vi "Frame Set Sound.vi"(8 "error in (no error)":errorcluster, 10 "Sound":string, 11 "IDE simple in":refnum<class "LF2R IDE.lvclass">) -> (0 "error out":errorcluster, 3 "IDE simple out":refnum<class "LF2R IDE.lvclass">)   [LabVIEW 2018, in "LF2R IDE.lvlib" / "LF2R IDE.lvclass"]
uses:
  LF2R IDE.lvclass
  LF2R IDE.lvclass/LF2R IDE.ctl
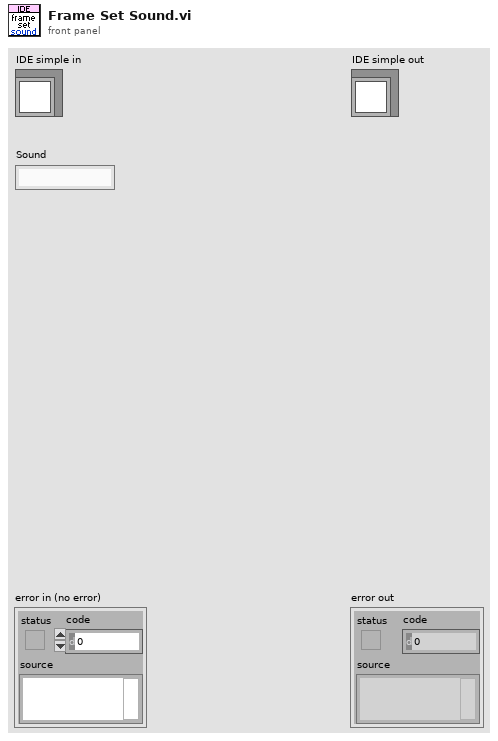
[diagram p1: front panel]
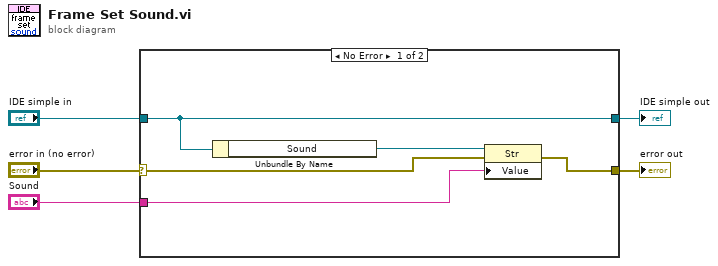
[diagram p0: block diagram]
diagram:
  n1 = case shown="No Error" "error in (no error)" {
    selector: "error in (no error)" -> [w6 w12]
    tunnel: [w7 w12] -> w4
    tunnel: [w10 w11] -> w2
    tunnel: "IDE simple in" -> [w10 w11]
    tunnel: "Sound" -> [w8 _]
    frame No Error {
      n2 = Unbundle By Name(w10) -> ("Sound"=w9:refnum<vi>)
      n3 = property class="Str"(reference=w9, error in=w6, "Value"=w8) -> (error out=w7:errorcluster)  [unwired: 1 out]
    }
    frame Error {
    }
  }
  "error out" <- w4
  "IDE simple out" <- w2
